vi "Parse Response.vi"(8 "error in (no error)":errorcluster, 10 "<JSON> Response":string, 11 "JSON-RPC in":refnum<class "JSON-RPC.lvclass">) -> (0 "error out":errorcluster, 1 "results":string, 3 "JSON-RPC out":refnum<class "JSON-RPC.lvclass">, 4 "IDs":string, 6 "Equal?":bool)   [LabVIEW 2019, in "JSON-RPC.lvclass"]
doc: "Parse a Response object to extract an object's <b>result</b>, and <b>id</b>.\n\nThe <b>result</b> datatype is a JSON object and will need further processing to convert to LabVIEW data. It is formatted in the same way as a Request object's params.\n\nhttps://www.jsonrpc.org/specification"
uses:
  JSON-RPC.lvclass
  JSON-RPC.lvclass/JSON-RPC.ctl
  private/Parse Response-JSONtext.vi/7ce7fba8-9f44-478d-b6cb-b571ff29f2f5.vi
  private/Parse Response-JSONtext.vi/8c905beb-ab4c-49e3-b5c6-2c663b7b30d7.vi
  private/Parse Response-JSONtext.vi/fce5892e-0c40-47e1-88e0-6c122aadefe2.vi
  <vilib>/JDP Science/JSONtext/Find Item.vi
  <vilib>/JDP Science/JSONtext/Next JSON Value.vi
  <vilib>/JDP Science/JSONtext/String Subset.vi
  <vilib>/JDP Science/JSONtext/Parsing/Advance past next JSON Value (inlined COPY).vi
  <vilib>/JDP Science/JSONtext/Parsing/Advance past whitespace.vi
  <vilib>/JDP Science/JSONtext/Parsing/Advance past String.vi
  <vilib>/JDP Science/JSONtext/Parsing/Advance past Number.vi
  <vilib>/JDP Science/JSONtext/Parsing/Advance past Line Ending.vi
  <vilib>/JDP Science/JSONtext/Get all Object Items.vi
  <vilib>/JDP Science/JSONtext/Parsing/Parse Full Path or Item Name.vi
  <vilib>/JDP Science/JSONtext/Parsing/Advance past Array.vi
  <vilib>/JDP Science/JSONtext/Parsing/Advance past Object.vi
  <vilib>/JDP Science/JSONtext/support/Error Cluster From Code.vi
  <vilib>/JDP Science/JSONtext/Offset/Find Item Locations by Path.vi
  <vilib>/JDP Science/JSONtext/JSON text to Variant.vi
  <vilib>/Utility/error.llb/Error Cluster From Error Code.vi
  <vilib>/JDP Science/JSONtext/LVClass Serializer/JSONtext LVClass Serializer.lvclass
  <vilib>/JDP Science/JSONtext/JSONtext.lvlib
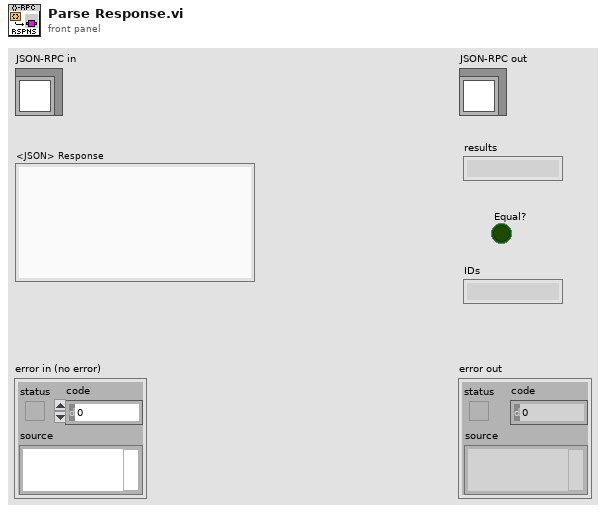
[diagram p1: front panel]
types:
  T1 = typedef "JSONtext.lvlib/JSON Value Type.ctl" = enum16{"Not a JSON Value", "JSON Object", "JSON Array", "String", "Number", "true", "false", "null"}
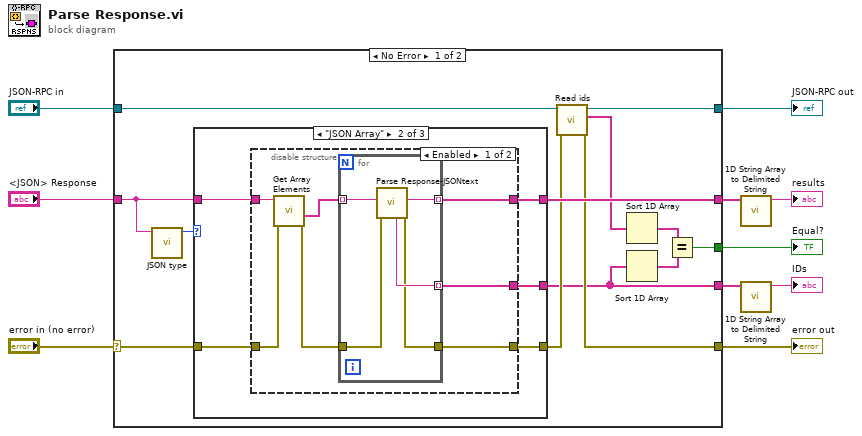
[diagram p0: block diagram]
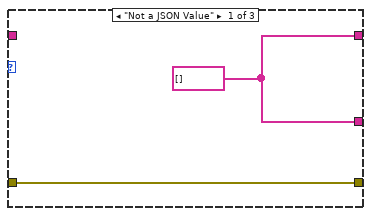
[diagram p2: hidden frame]
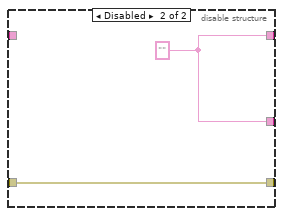
[diagram p3: hidden frame]
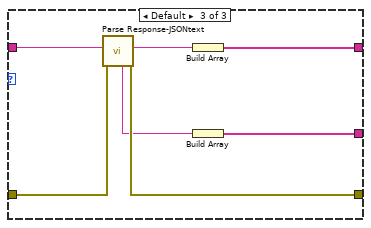
[diagram p4: hidden frame]
diagram:
  n1 = case shown="No Error" "error in (no error)" {
    selector: "error in (no error)" -> [w21 w53]
    tunnel: [w16 w53] -> w9
    tunnel: "JSON-RPC in" -> [w18 w52]
    tunnel: "<JSON> Response" -> [w22 _]
    tunnel: [w19 w52] -> w6
    tunnel: [w20 _] -> w2
    tunnel: [w15 _] -> w5
    tunnel: [w13 _] -> w4
    frame No Error {
      n2 = call <vilib>:"JSON type.vi"("JSON"=w22) -> ("JSON Value Type"=w23:T1)  [unwired: 9 in, 1 out]
      n3 = case shown="\"JSON Array\"" w23 {
        tunnel: w21 -> [w25 w27 w50]
        tunnel: [w25 w30 w49] -> w17
        tunnel: w22 -> [_ w28 w51]
        tunnel: [w24 w29 w47] -> w20
        tunnel: [w24 w26 w45] -> w13
        frame "Not a JSON Value" {
          w24 = string[] []
        }
        frame "JSON Array" {
          n4 = disable-structure shown="Enabled" {
            disable-tunnel: [w37 w43] -> w30
            disable-tunnel: [w31 w44] -> w29
            disable-tunnel: w28 -> [w36 _]
            disable-tunnel: w27 -> [w35 w43]
            disable-tunnel: [w32 w44] -> w26
            frame Enabled {
              n5 = call <vilib>:"Get Array Elements.vi"("error in (no error)"=w35, "JSON"=w36) -> ("error out"=w33:errorcluster, "<JSON>"=w34:string[])  [unwired: 7 in, 1 out]
              n6 = for {
                tunnel: w34 -> [w42] mode=indexing
                tunnel: [w40] -> w31 mode=indexing
                tunnel: [w39] -> w32 mode=indexing
                tunnel: w33 -> [w41]
                tunnel: [w38] -> w37
                n7 = call "Parse Response-JSONtext.vi"("error in (no error)"=w41, "<JSON> Response"=w42) -> ("error out"=w38:errorcluster, "result"=w40:string, "id"=w39:string)  [unwired: 7 in]
              }
            }
            frame Disabled {
              w44 = ""
            }
          }
        }
        frame Default {
          n8 = call "Parse Response-JSONtext.vi"("error in (no error)"=w50, "<JSON> Response"=w51) -> ("error out"=w49:errorcluster, "result"=w48:string, "id"=w46:string)  [unwired: 7 in]
          n9 = Build Array(w48) -> (w47:string[])
          n10 = Build Array(w46) -> (w45:string[])
        }
      }
      n11 = call "Read ids.vi"("error in (no error)"=w17, "JSON-RPC in"=w18) -> ("error out"=w16:errorcluster, "ids"=w14:string[], "JSON-RPC out"=w19:refnum<class "JSON-RPC.lvclass">)  [unwired: 7 in]
      n12 = Sort 1D Array(array=w14) -> (sorted array=w12:string[])
      n13 = Sort 1D Array(array=w13) -> (sorted array=w11:string[])
      n14 = Equal?(x=w12, y=w11) -> (x = y?=w15:bool)
    }
    frame Error {
    }
  }
  "error out" <- w9
  "JSON-RPC out" <- w6
  "Equal?" <- w5
  n15 = call <vilib>:"1D String Array to Delimited String.vi"("string array"=w2) -> ("delimited string"=→"results":string)  [unwired: 10 in]
  n16 = call <vilib>:"1D String Array to Delimited String.vi"("string array"=w4) -> ("delimited string"=→"IDs":string)  [unwired: 10 in]
